vi "Override Error.vi"(10 "Error":errorcluster, 11 "Base Event in":refnum<class "Base Event.lvclass">) -> (3 "Base Event out":refnum<class "Base Event.lvclass">)   [LabVIEW 2021, in "jettl.lvlib" / "Base Event.lvlib" / "Base Event.lvclass"]
uses:
  Base Event.lvclass
  Base Event.lvclass/Base Event.ctl
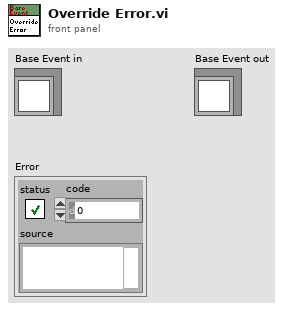
[diagram p1: front panel]
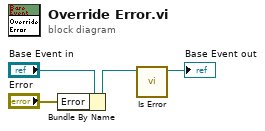
[diagram p0: block diagram]
diagram:
  n1 = Bundle By Name(cluster="Base Event in", "Error"="Error") -> (w2:refnum<class "Base Event.lvclass">)
  n2 = call "Is Error.vi"("Base Event jettl in"=w2) -> ("Base Event jettl out"=→"Base Event out":refnum<class "Base Event.lvclass">)  [unwired: 10 in]
